vi "Set state.vi"(5 "countLimit":u32, 7 "timeLimit":u32, 8 "error in (no error)":errorcluster, 10 "newState":i32=-1, 11 "StateManager in":refnum<class "StateManager.lvclass">) -> (0 "error out":errorcluster, 3 "StateManager out":refnum<class "StateManager.lvclass">)   [LabVIEW 2018, in "StateManager.lvclass"]
uses:
  StateManager.lvclass
  StateManager.lvclass/StateManager.ctl
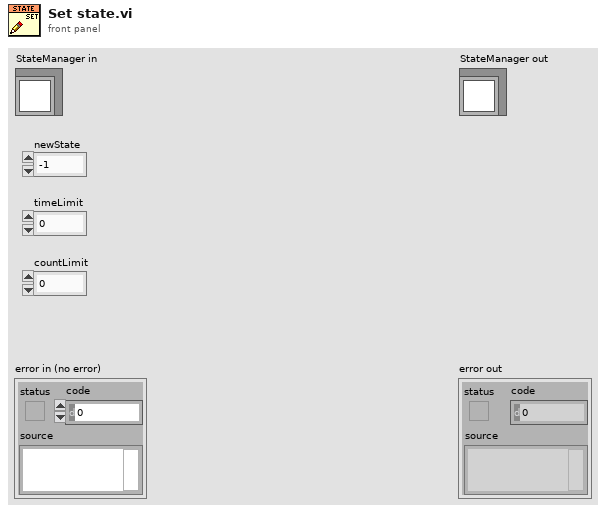
[diagram p1: front panel]
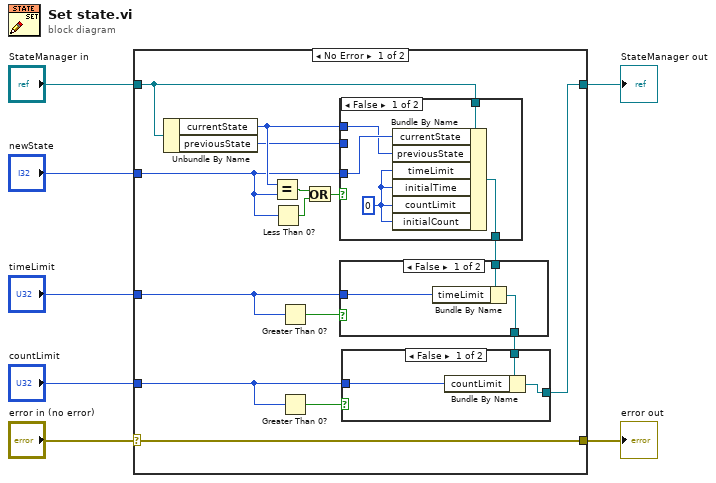
[diagram p0: block diagram]
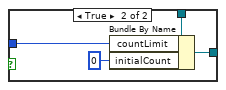
[diagram p2: hidden frame]
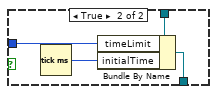
[diagram p3: hidden frame]
diagram:
  n1 = case shown="No Error" "error in (no error)" {
    selector: "error in (no error)" -> [w22 w43]
    tunnel: [w22 w43] -> w6
    tunnel: [w13 w44] -> w5
    tunnel: "StateManager in" -> [w12 w44]
    tunnel: "newState" -> [w8 _]
    tunnel: "timeLimit" -> [w18 _]
    tunnel: "countLimit" -> [w14 _]
    frame No Error {
      n2 = Unbundle By Name(w12) -> ("currentState"=w21:u32, "previousState"=w20:u32)
      n3 = Equal?(x=w21, y=w8) -> (x = y?=w10:bool)
      n4 = Less Than 0?(x=w8) -> (x < 0?=w9:bool)
      n5 = Greater Than 0?(x=w18) -> (x > 0?=w19:bool)
      n6 = Greater Than 0?(x=w14) -> (x > 0?=w15:bool)
      n7 = Or(x=w10, y=w9) -> (x .or. y?=w11:bool)
      n8 = case shown="False" w11 {
        tunnel: w21 -> [w39 _]
        tunnel: w20 -> [_ _]
        tunnel: w8 -> [w40 _]
        tunnel: w12 -> [w41 w42]
        tunnel: [w38 w42] -> w17
        frame False {
          w37 = u32 0 ("initialCount")
          n9 = Bundle By Name(cluster=w41, "currentState"=w40, "previousState"=w39, "timeLimit"=w37, "initialTime"=w37, "countLimit"=w37, "initialCount"=w37) -> (w38:refnum<class "StateManager.lvclass">)
        }
        frame True {
        }
      }
      n10 = case shown="False" w19 {
        tunnel: w18 -> [w30 w36]
        tunnel: w17 -> [w32 w35]
        tunnel: [w31 w34] -> w16
        frame False {
          n11 = Bundle By Name(cluster=w32, "timeLimit"=w30) -> (w31:refnum<class "StateManager.lvclass">)
        }
        frame True {
          n12 = Tick Count (ms)() -> (millisecond timer value=w33:u32)
          n13 = Bundle By Name(cluster=w35, "timeLimit"=w36, "initialTime"=w33) -> (w34:refnum<class "StateManager.lvclass">)
        }
      }
      n14 = case shown="False" w15 {
        tunnel: w14 -> [w25 w29]
        tunnel: w16 -> [w23 w28]
        tunnel: [w24 w27] -> w13
        frame False {
          n15 = Bundle By Name(cluster=w23, "countLimit"=w25) -> (w24:refnum<class "StateManager.lvclass">)
        }
        frame True {
          n16 = Bundle By Name(cluster=w28, "countLimit"=w29, "initialCount"=u32 0) -> (w27:refnum<class "StateManager.lvclass">)
        }
      }
    }
    frame Error {
    }
  }
  "error out" <- w6
  "StateManager out" <- w5
